vi "Read Msg Output.vi"(11 "Stop Msg Output in":refnum<class "Stop Msg Output.lvclass">) -> ()   [LabVIEW 2020, in "jettl.lvlib" / "Stop jettl Msg.lvlib" / "Stop Msg Output.lvlib" / "Stop Msg Output.lvclass"]
uses:
  Stop Msg Output.lvclass
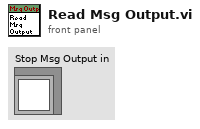
[diagram p1: front panel]
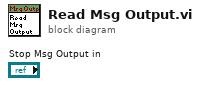
[diagram p0: block diagram]
diagram:
